vi "Example Read Callback.vi"() -> ()   [LabVIEW 2013]
uses:
  C:/tf/play/labview/Tinkerforge.dll
  Tinkerforge.dll
panel:
  out "data":u8[](array[numeric])
  out "identifier":i64
  out "frameType":u8
  in  "stop":bool
  in  "uid":string="5556"
  in  "port":i32=4223
  in  "host":string="localhost"
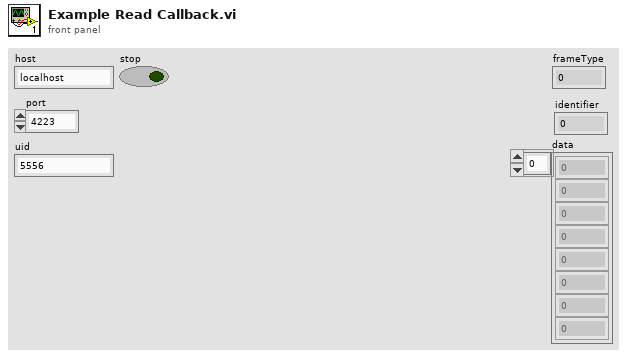
[diagram p1: front panel]
types:
  T1 = cluster{"data":u8[], "frameType":u8, "identifier":i64}
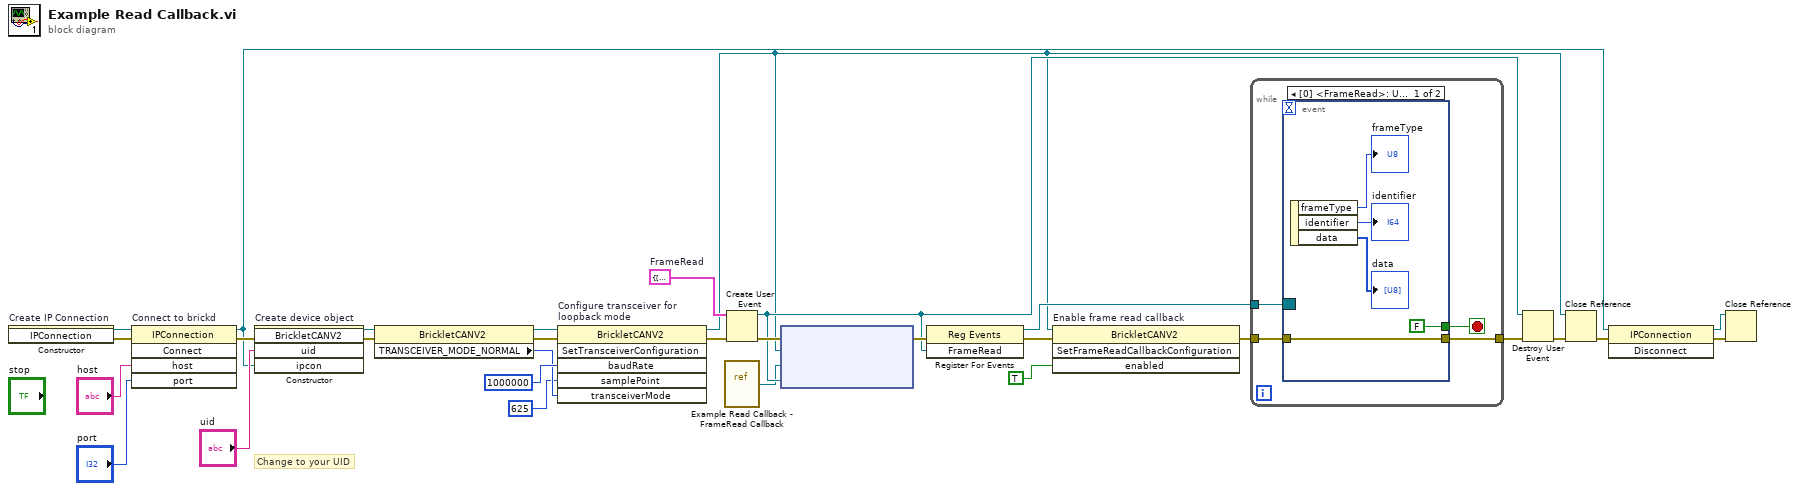
[diagram p0: block diagram]
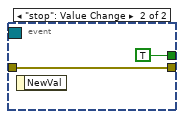
[diagram p2: hidden frame]
diagram:
  w14 = T1 {"data"=[], "frameType"=0, "identifier"=0}  # FrameRead
  # "Change to your UID"
  n1 = constructor on="Create IP Connection" class="IPConnection"() -> (reference out=w30:refnum<k24>, error out=w15:errorcluster)  [unwired: 3 in, 1 out]
  n2 = invoke on="Connect to brickd" class="IPConnection" method="Connect"(reference=w30, error in=w15, "host"="host", "port"="port") -> (reference out=w23:refnum<k24>, error out=w26:errorcluster)  [unwired: 1 in, 3 out]
  n3 = constructor on="Create device object" class="BrickletCANV2"(error in=w26, "uid"="uid", "ipcon"=w23) -> (reference out=w11:refnum<k24>, error out=w12:errorcluster)  [unwired: 2 in, 3 out]
  n4 = property class="BrickletCANV2"(reference=w11, error in=w12) -> (reference out=w7:refnum<k24>, error out=w8:errorcluster, "TRANSCEIVER_MODE_NORMAL"=w3:u8)
  n5 = invoke on="Configure transceiver for\nloopback mode" class="BrickletCANV2" method="SetTransceiverConfiguration"(reference=w7, error in=w8, "baudRate"=i64 1000000, "samplePoint"=625, "transceiverMode"=w3) -> (reference out=w10:refnum<k24>, error out=w9:errorcluster)  [unwired: 1 in, 4 out]
  n6 = vi-ref "Example Read Callback - FrameRead Callback.vi"() -> ("vi reference"=w5:refnum<vi>)
  n7 = Create User Event(user event datatype=w14, error in=w9) -> (user event=w17:refnum<user-event>, error out=w21:errorcluster)
  n8 = node ("Register Event Callback")(w21, w10, w5, w17) -> (w20:errorcluster)  [unwired: 1 in, 1 out]
  n9 = register-events(error in=w20, w17) -> (reference out=w19:refnum<event-registration>, error out=w13:errorcluster)  [unwired: 1 in]
  n10 = invoke on="Enable frame read callback" class="BrickletCANV2" method="SetFrameReadCallbackConfiguration"(reference=w10, error in=w13, "enabled"=TRUE) -> (error out=w1:errorcluster)  [unwired: 1 in, 3 out]
  n11 = while {
    tunnel: w19 -> [w34]
    tunnel: [w33] -> w18
    tunnel: w1 -> [w32]
    stop <- w31 stop-if-true
    n12 = event shown="[0] <FrameRead>: User Event" {
      selector: w34 -> [_ _]
      dyn-events: _ -> [_ _]
      timeout: _ -> [_ _]
      tunnel: [w39 w40] -> w33
      tunnel: w32 -> [w39 w40]
      tunnel: [FALSE TRUE] -> w31
      event User Event {
        n13 = event-data() -> ("frameType"=→"frameType":u8, "identifier"=→"identifier":i64, "data"=→"data":u8[])  [unwired: 1 in]
      }
      event "stop": Value Change {
        n14 = event-data() -> ()  [unwired: 1 in, 1 out]
      }
    }
  }
  n15 = Destroy User Event(user event=w17, error in=w18) -> (error out=w16:errorcluster)
  n16 = Close Reference(reference=w10, error in (no error)=w16) -> (error out=w25:errorcluster)
  n17 = invoke class="IPConnection" method="Disconnect"(reference=w23, error in=w25) -> (reference out=w22:refnum<k24>, error out=w24:errorcluster)  [unwired: 1 in, 1 out]
  n18 = Close Reference(reference=w22, error in (no error)=w24) -> ()  [unwired: 1 out]
